vi "系统设置全局变量.vi"() -> ()   [LabVIEW 2016]
panel:
  in  "站点名称":string
  in  "旁路系统启用":bool
  in  "VI名称":string
  in  "综合生物毒性启用":bool
  in  "雷达流速仪启用":bool
  in  "ADCP启用":bool
  out "流程测试中":bool
  in  "性能测试模式":bool
  in  "挥发酚启用":bool
  in  "采配水运行间隔":i16 min=0 max=24
  in  "重金属启用":bool
  out "24H周期设置":bool[](array[boolean])
  out "启用运维打卡":bool caption="启用"
  in  "氟化物启用":bool
  in  "加标回收模块版本":T1=enum."V4"
  in  "多参数模块版本":T2=enum."集成式多参"
  in  "总氮模块版本":T3=enum."V3"
  in  "总磷模块版本":T3=enum."V3"
  in  "氨氮模块版本":T3=enum."V3"
  out "进样类型":T4={"氨氮采样杯采样"=TRUE, "总磷采样杯采样"=TRUE, "总氮采样杯采样"=TRUE, "CODMn采样杯采样"=TRUE, "CODcr采样杯采样"=TRUE, "氟化物采样杯采样"=TRUE, "挥发酚采样杯采样"=TRUE}
  in  "CODcr模块版本":T5
  in  "设备类型":T6
  in  "采配水模块类型":T7=enum."V4"
  in  "CODMn模块版本":T8
  in  "SYSTEM Interface.总磷总氮类型":T9=enum."总磷总氮二合一模块"
  in  "采水模式":enum16{"单采水点", "交替采水"}(ring)
  in  "权限密码":u32[](array[numeric])=[0, 23506, 783523506, 783523103]
  in  "温湿度报警":T10={"温度报警"=50, "湿度报警"=98, "报警确认时间"=120, "布尔"=FALSE} {"报警确认时间" format="%02.0f"; "湿度报警" format="%02.0f"; "温度报警" format="%02.0f"}
  in  "多参数运行间隔":i16=4 min=1 max=24
  in  "总氮启用":bool caption="总磷总氮禁用"
  in  "站点系列号":string
  in  "自动运行启动参数":T11
  in  "系统重启设置":T12 {"分" max=59 format="%02.0f"; "时" max=23 format="%02.0f"}
  in  "首页显示信息设置":T13={"水温"=TRUE, "pH"=FALSE, "DO"=FALSE, "Cond"=FALSE, "Turb"=FALSE, "氨氮"=FALSE, "总磷"=FALSE, "总氮"=FALSE, "CODMn"=FALSE, "CODCr"=FALSE, "水位"=FALSE, "流速"=FALSE, "瞬时流量"=FALSE, "ORP"=FALSE, "氟化物"=FALSE, "铅"=FALSE, "镉"=FALSE, "铜"=FALSE, "锌"=FALSE, "汞"=FALSE, "叶绿素a"=FALSE, "藻密度"=FALSE, "氯化物"=FALSE, "挥发酚"=FALSE, "盐度"=FALSE, "磷酸盐"=FALSE, "硝氮"=FALSE, "亚硝氮"=FALSE, "硅酸盐"=FALSE, "硫化物"=FALSE, "余氯"=FALSE}
  in  "流量阈值":dbl=4.0 min=1.0 max=24.0
  in  "时间阈值":u16=4 min=1 max=24
  in  "超标留样启用":bool caption="采配水禁用"
  in  "周期设置":enum16{"自由设定", "国标协议", "流量设定"}(ring)
  in  "运行间隔":i16=4 min=1 max=24
  in  "跨度核查时间":u16(ring)=6 items=["00H", "01H", "02H", "03H", "04H", "05H", "06H", "07H", "08H", "09H", "10H", "11H", "12H", "13H", "14H", "15H", "16H", "17H", "18H", "19H", "20H", "21H", "22H", "23H"]
  in  "空白核查时间":u16(ring)=2 items=["00H", "01H", "02H", "03H", "04H", "05H", "06H", "07H", "08H", "09H", "10H", "11H", "12H", "13H", "14H", "15H", "16H", "17H", "18H", "19H", "20H", "21H", "22H", "23H"]
  in  "质控启动日期":string(combo)="关闭"
  in  "运行模式":enum16{"维护模式", "常规模式", "应急模式", "质控模式"}(ring)
  in  "多参数启用":bool caption="多参数禁用"
  in  "其他启用":bool caption="其他禁用"
  in  "河水净化启用":bool caption="电源管理禁用"
  in  "流量计启用":bool caption="流量计禁用"
  in  "质控单元启用":bool caption="质控单元禁用"
  in  "总磷总氮启用":bool caption="总磷总氮禁用"
  in  "氨氮启用":bool caption="氨氮禁用"
  in  "CODcr启用":bool caption="CODcr禁用"
  in  "CODMn启用":bool caption="CODMn禁用"
  in  "采配水启用":bool caption="采配水禁用"
  # "质控频次："
  # "空白核查时间："
  # "跨度核查时间："
  # "频次："
  # "时间："
  # "："
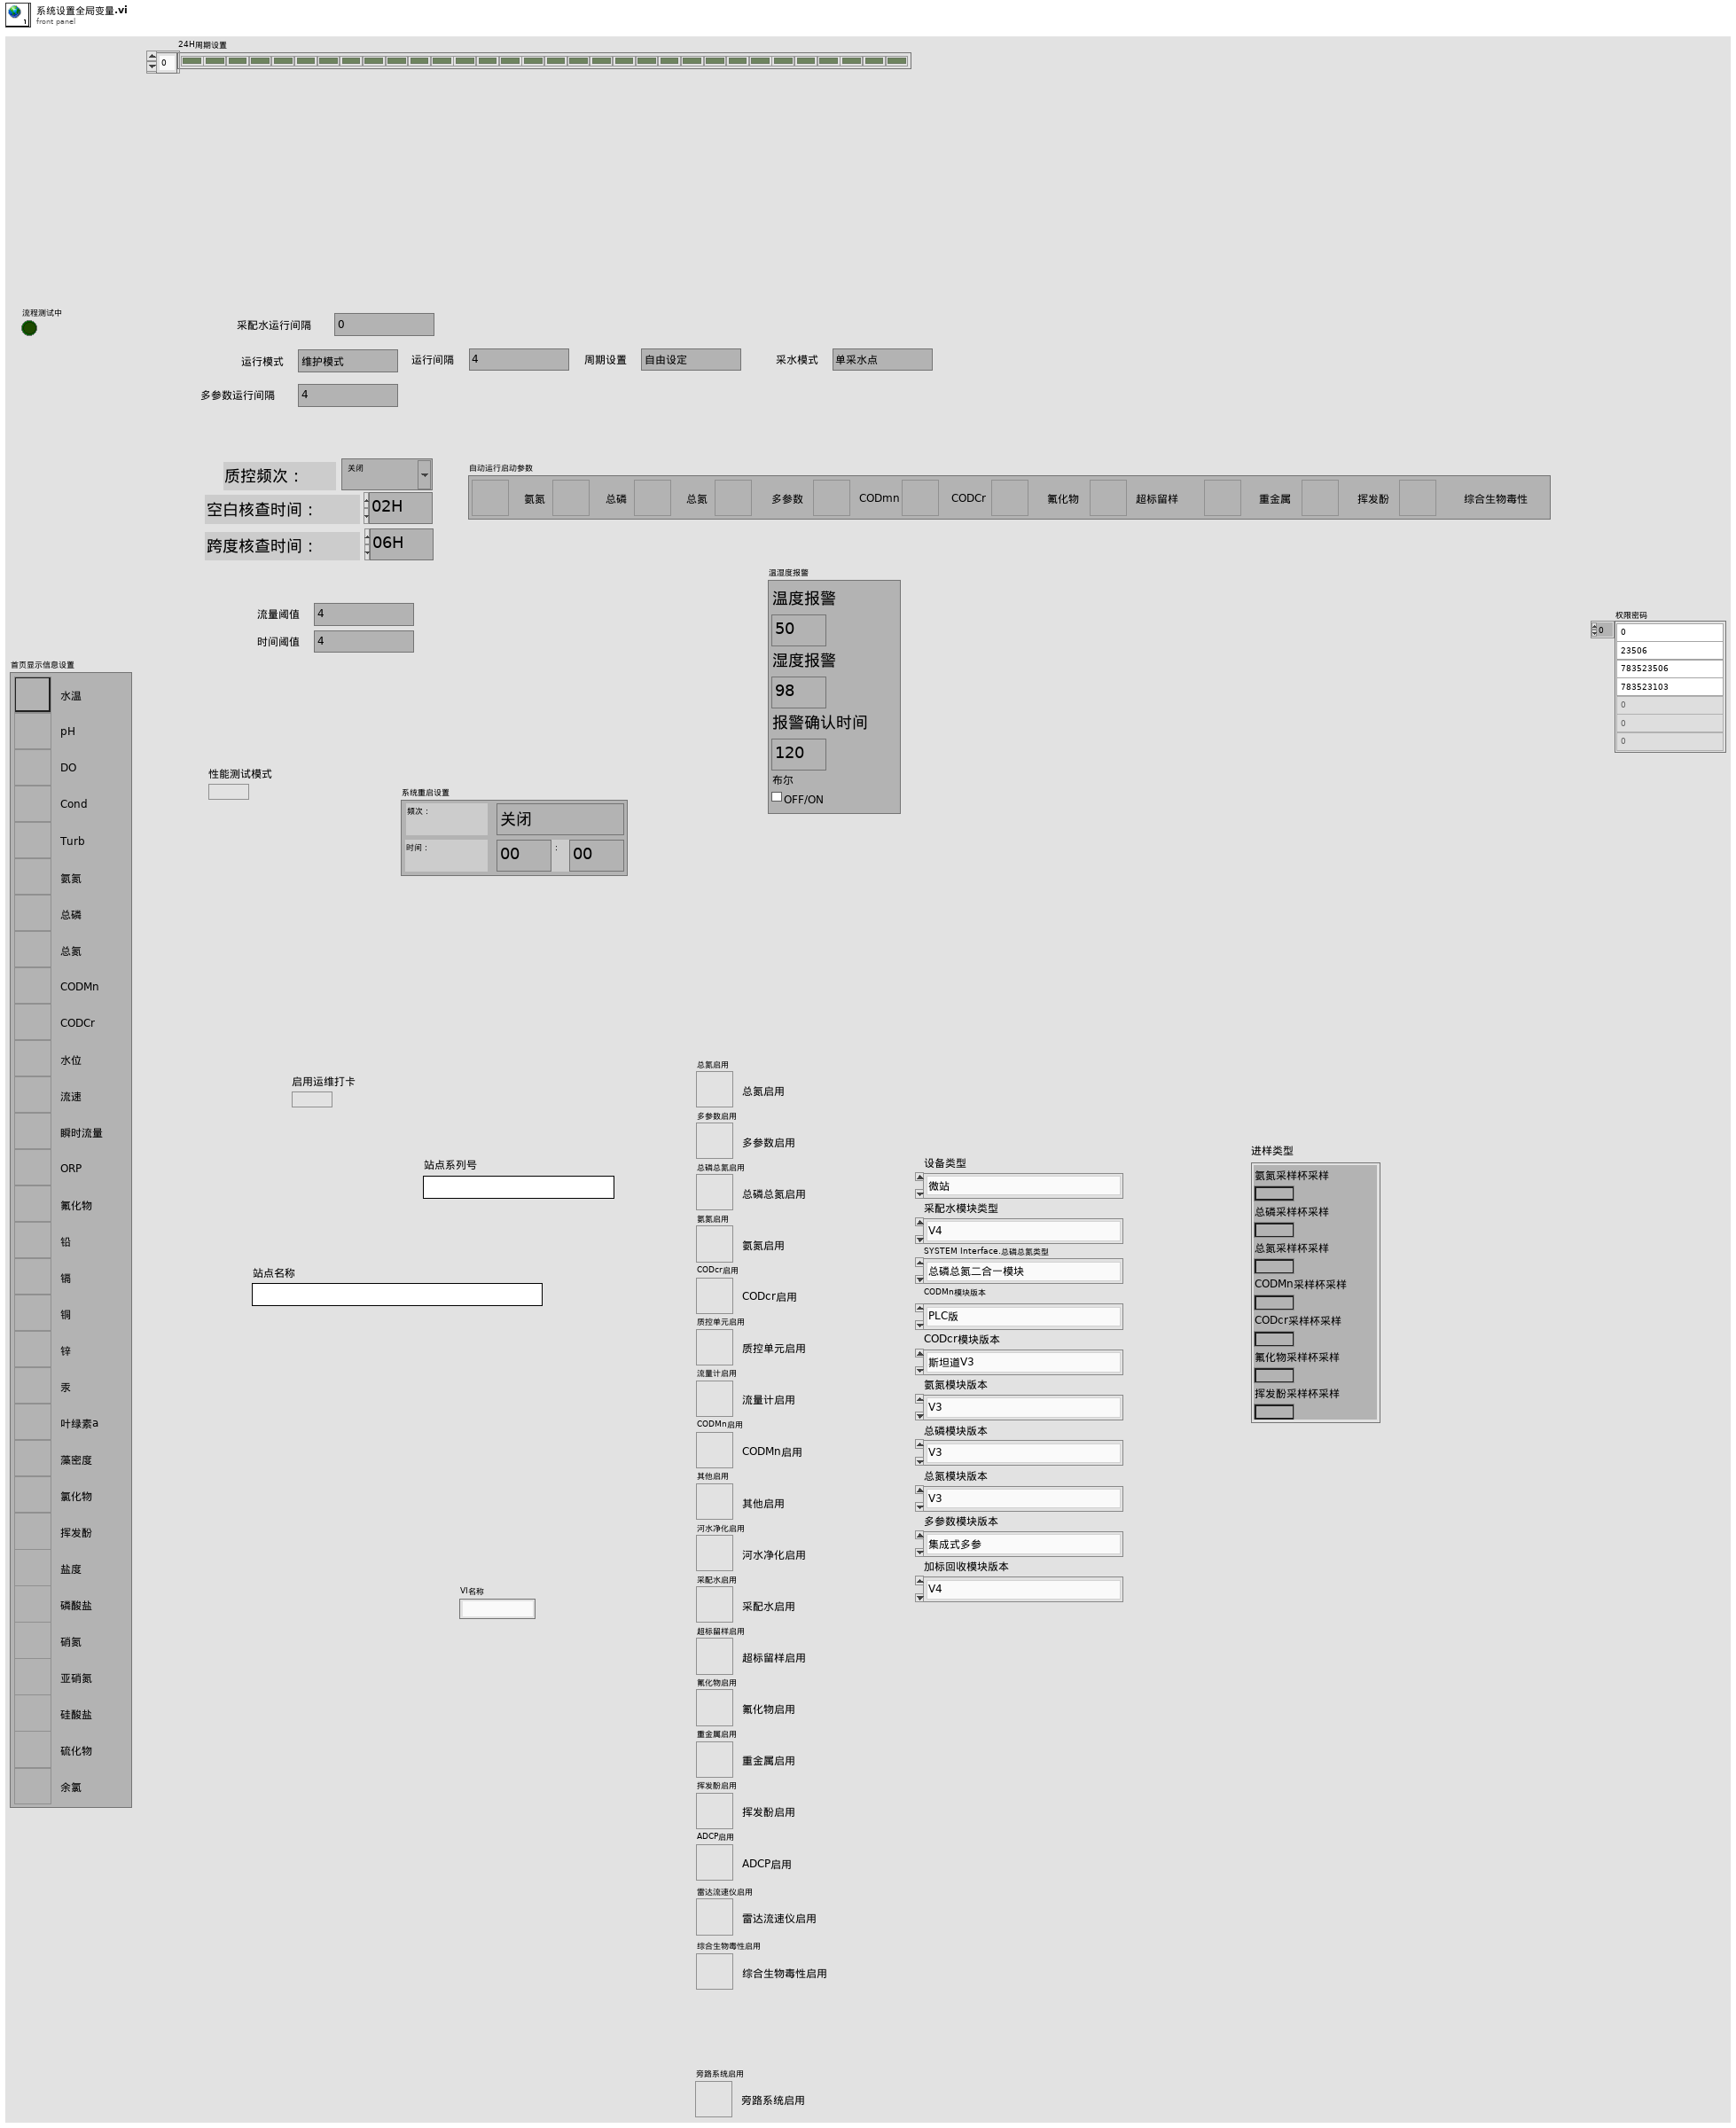
[diagram p1: front panel]
types:
  T1 = typedef "加标回收模块版本.ctl" = enum16{"V1", "V2", "V4"}
  T2 = typedef "多参数模块版本.ctl" = enum16{"原位多参数", "集成式多参"}
  T3 = typedef "氨氮总磷总氮模块版本.ctl" = enum16{"V2", "V3"}
  T4 = cluster{"氨氮采样杯采样":bool, "总磷采样杯采样":bool, "总氮采样杯采样":bool, "CODMn采样杯采样":bool, "CODcr采样杯采样":bool, "氟化物采样杯采样":bool, "挥发酚采样杯采样":bool}
  T5 = typedef "CODcr模块版本.ctl" = enum16{"斯坦道V3", "点创"}
  T6 = typedef "设备类型.ctl" = enum16{"微站", "固定站", "浮船"}
  T7 = typedef "采配水类型.ctl" = enum16{"V1", "V2", "V3", "V4", "室内V1", "室内V2", "固定站V1", "固定站V2", "浮船V1", "浮船V2", "养殖尾水", "广东华南所"}
  T8 = typedef "CODMn模块版本.ctl" = enum16{"PLC版", "单片机版", "通用流路版本"}
  T9 = typedef "模块配置类型.ctl" = enum16{"单模块", "总磷总氮二合一模块", "氨氮总磷二合一模块"}
  T10 = cluster{"温度报警":u16, "湿度报警":u16, "报警确认时间":u16, "布尔":bool}
  T11 = typedef "启动参数.ctl" = cluster{"氨氮":bool, "总磷":bool, "总氮":bool, "多参数":bool, "CODmn":bool, "CODCr":bool, "氟化物":bool, "超标留样":bool, "重金属":bool, "挥发酚":bool, "综合生物毒性":bool}
  T12 = cluster{"频次":enum16{"关闭", "每天", "星期一", "星期二", "星期三", "星期四", "星期五", "星期六", "星期日"}, "时":u16, "分":u16}
  T13 = cluster{"水温":bool, "pH":bool, "DO":bool, "Cond":bool, "Turb":bool, "氨氮":bool, "总磷":bool, "总氮":bool, "CODMn":bool, "CODCr":bool, "水位":bool, "流速":bool, "瞬时流量":bool, "ORP":bool, "氟化物":bool, "铅":bool, "镉":bool, "铜":bool, "锌":bool, "汞":bool, "叶绿素a":bool, "藻密度":bool, "氯化物":bool, "挥发酚":bool, "盐度":bool, "磷酸盐":bool, "硝氮":bool, "亚硝氮":bool, "硅酸盐":bool, "硫化物":bool, "余氯":bool}
diagram:
